vi "Rotate.vi"(8 "error in":errorcluster, 9 "Rotate":dbl format="%#_13g", 10 "Input Point":T1 {"Y" format="%.2f"; "X" format="%.2f"}, 11 "Rotation center Point":T1 {"Y" format="%.2f"; "X" format="%.2f"}) -> (0 "error out":errorcluster, 3 "Output Point":cluster{"X":dbl, "Y":dbl})   [LabVIEW 2015]
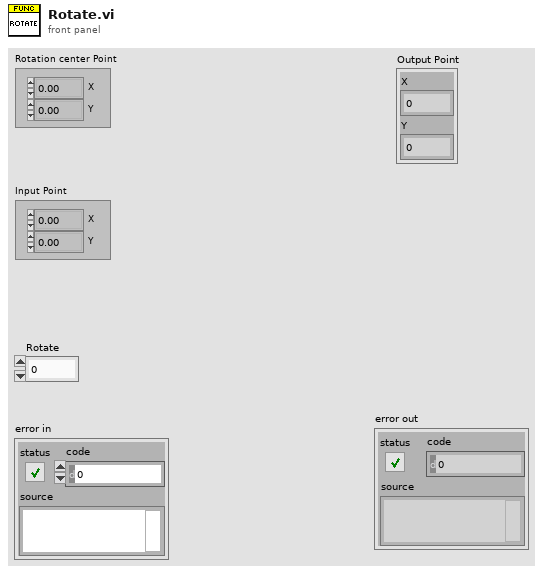
[diagram p1: front panel]
types:
  T1 = typedef "IMAQ Point" = cluster{"X":sgl, "Y":sgl}
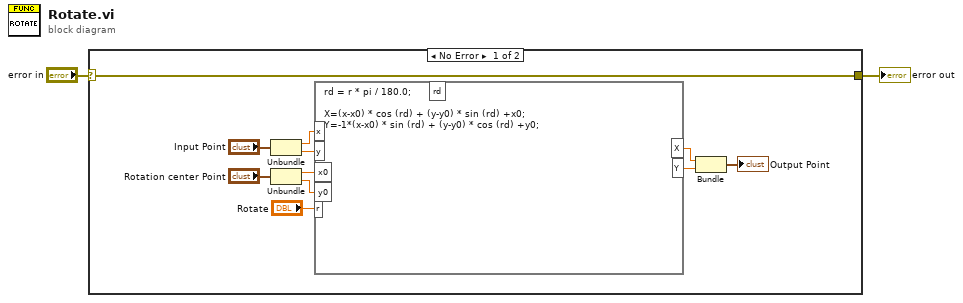
[diagram p0: block diagram]
diagram:
  n1 = case shown="No Error" "error in" {
    selector: "error in" -> [w3 w14]
    tunnel: [w3 w14] -> w1
    frame No Error {
      n2 = Unbundle("Input Point") -> ("X"=w9:sgl, "Y"=w6:sgl)
      n3 = Unbundle("Rotation center Point") -> ("X"=w8:sgl, "Y"=w7:sgl)
      n4 = formula code="rd = r * pi / 180.0;\n\nX=(x-x0) * cos (rd) + (y-y0) * sin (rd) +x0;\nY=-1*(x-x0) * sin (rd) + (y-y0) * cos (rd) +y0;"("r"="Rotate", "x0"=w8, "y0"=w7, "x"=w9, "y"=w6) -> ("X"=w13:dbl, "Y"=w12:dbl)  [unwired: 1 out]
      n5 = Bundle("X"=w13, "Y"=w12) -> (→"Output Point":cluster{"X":dbl, "Y":dbl})  [unwired: 1 in]
    }
    frame Error {
    }
  }
  "error out" <- w1
